vi "add.VI"(9 "数值 2":dbl, 11 "数值":dbl) -> (3 "数值 3":dbl)   [LabVIEW 2018]
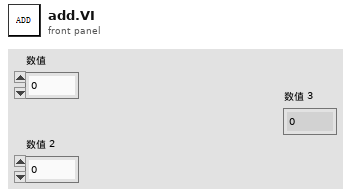
[diagram p1: front panel]
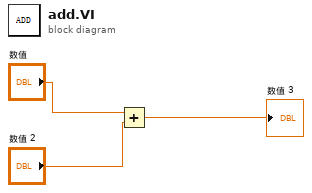
[diagram p0: block diagram]
diagram:
  n1 = Add(x="数值", y="数值 2") -> (x+y=→"数值 3":dbl)
